vi "NI_Read XLSX File (revised, faster).vi"(4 "Remove empty rows":bool, 6 "Remove empty columns":bool, 8 "error in":errorcluster, 9 "Repeat multicell values":bool, 11 "XLSX File":path) -> (0 "error out":errorcluster, 2 "Sheet Names":string[](array[string]), 3 "Sheet Data":cluster{"Array":string[][]}[](array[cluster]))   [LabVIEW 2021, in "Files.lvlib"]
doc: "Reads all sheets from the specified <b>XLSX File</b>. This VI does <b>not</b> require Microsoft Excel to be installed.\n\nEach sheet is returned as a 2D Array of Strings. You will need to perform additional conversion if you require data in numeric format.\n\nTime data (date and/or time) is returned as a number of days elapsed since January 1, 1900. Hour/minute/second information will be returned as a fraction of a day (24 hours).\n\nAdded: option to fill table with repeated values to reflect multicell-spanning super-cells"
uses:
  Files.lvlib
  <vilib>/zip/NI_Unzip.lvlib
panel:
  out "UnDot?":bool
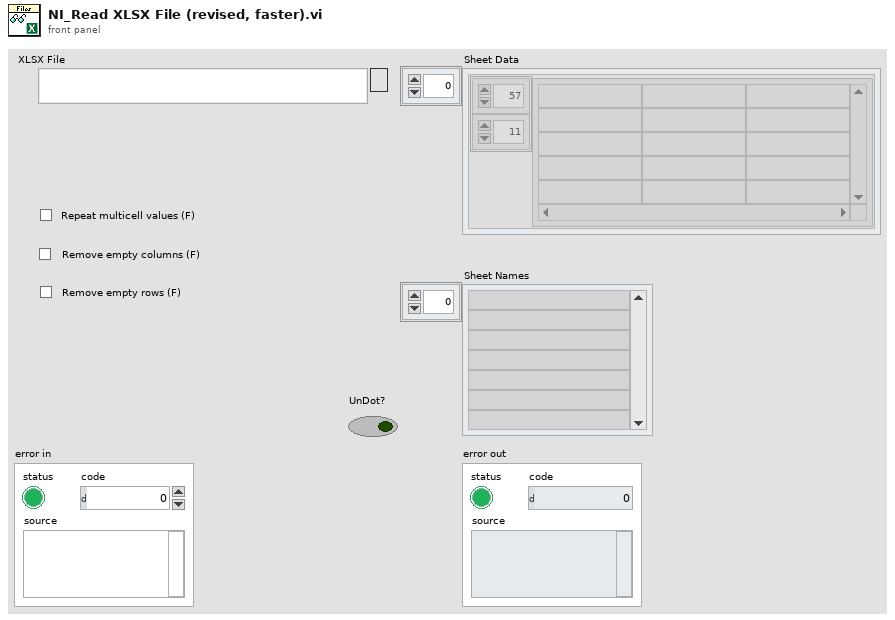
[diagram p1: front panel]
types:
  T1 = cluster{"Top Left Row":i32, "Top Left Col":i32, "Bottom Right Row":i32, "Bottom Right Col":i32}[]
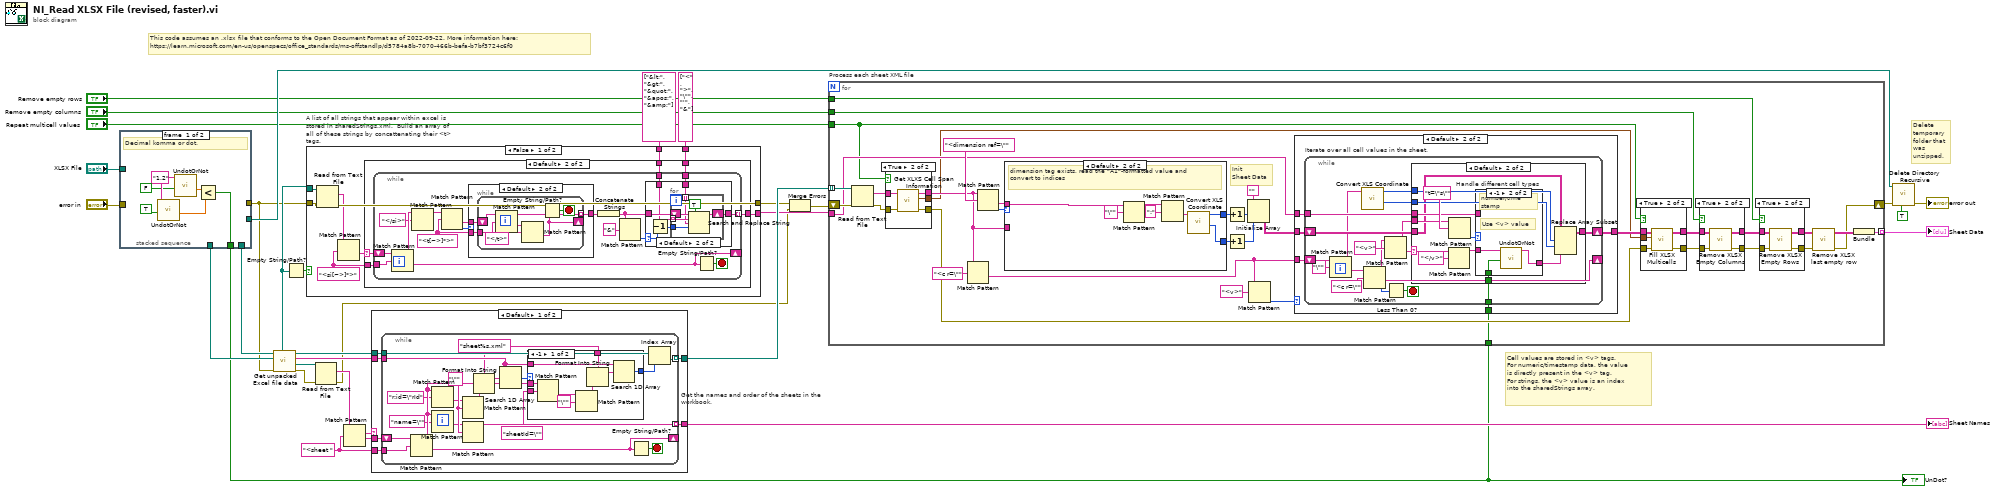
[diagram p0: block diagram]
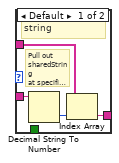
[diagram p8: hidden frame]
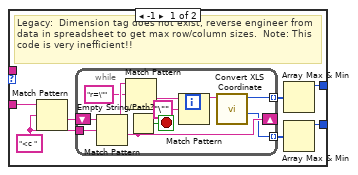
[diagram p9: hidden frame]
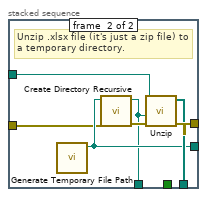
[diagram p16: hidden frame]
diagram:
  w27 = "<sheet "
  # "Cell values are stored in <v> tags.\nFor numeric/timestamp data, the value\nis directly present in the <v> tag.\nFor strings, the <v> value is an index\ninto the sharedStrings array."
  # "Delete temporary folder that was unzipped."
  # "This code assumes an .xlsx file that conforms to the Open Document Format as of 2022-09-22. More information here:\nhttps://learn.microsoft.com/en-us/openspecs/office_standards/ms-offstandlp/d5784a8b-7070-466b-befa-b7bf3724c6f0"
  n1 = stacked-sequence {
    tunnel: [_ w44] -> w4
    tunnel: [_ w43] -> w24
    tunnel: [_ w42] -> w31
    tunnel: [_ w41] -> w25
    tunnel: [w35 _] -> w10
    tunnel: "error in" -> [_ w40]
    tunnel: "XLSX File" -> [_ w39]
    frame #0 {
      w38 = "1.2" ("DottedNumber")
      # "Decimal komma or dot."
      n2 = call "UndotOrNot.vi"("UnDot?"=TRUE, "DottedNumber"=w38) -> ("Number"=w36:dbl)  [unwired: 8 in, 1 out]
      n3 = call "UndotOrNot.vi"("UnDot?"=FALSE, "DottedNumber"=w38) -> ("Number"=w37:dbl)  [unwired: 8 in, 1 out]
      n4 = Less?(x=w37, y=w36) -> (x < y?=w35:bool)
    }
    frame #1 {
      # "Unzip .xlsx file (it's just a zip file) to a temporary directory."
      n5 = call <vilib>:"Generate Temporary File Path.vi"() -> ("Unique Temporary File Path"=w42:path)  [unwired: 10 in, 1 out]
      n6 = call <vilib>:"Create Directory Recursive.vi"("error in (no error)"=w40, "directory"=w42) -> ("error out"=w45:errorcluster, "directory copy"=w41:path)  [unwired: 3 in, 1 out]
      n7 = call <vilib>:"Unzip.vi"("error in (no error)"=w45, "Target directory (same as Zip file if empty)"=w41, "Zip file"=w39) -> ("error out"=w44:errorcluster, "Unzipped files"=w43:path[])  [unwired: 6 in, 1 out]
    }
  }
  "UnDot?" <- w10
  n8 = call "Get unpacked Excel file data.vi"("Error In"=w4, "temp zip path"=w25, "Unzipped files"=w24) -> ("Error Out"=w3:errorcluster, "workbook.xml path"=w5:path, "sheet file names"=w6:string[], "sheet paths"=w26:path[], "sharedStrings path"=w15:path)  [unwired: 4 in]
  n9 = Empty String/Path?(string/path=w15) -> (empty?=w16:bool)
  n10 = case "A list of all strings that appear within excel is stored in sharedStrings.xml.  Build an array of all of these strings by concattenating their <t> tags." shown="False" w16 {
    tunnel: w4 -> [w54 w100]
    tunnel: [w52 w100] -> w18
    tunnel: w15 -> [w53 _]
    tunnel: [w51 _] -> w17
    tunnel: string[] ["&lt;", "&gt;", "&quot;", "&apos;", "&amp;"] -> [w47 _]
    tunnel: string[] ["<", ">", "\"", "'", "&"] -> [w46 _]
    frame False {
      w49 = "<si[~>]*>" ("regular expression")
      n11 = Read from Text File(file (use dialog)=w53, error in=w54) -> (text=w48:string, error out=w52:errorcluster)  [unwired: 2 in, 2 out]
      n12 = Match Pattern(string=w48, regular expression=w49) -> (after substring=w50:string)  [unwired: 1 in, 3 out]
      n13 = case shown="Default" w50 {
        selector: w50 -> [_ w57]
        tunnel: [_ w59] -> w51
        tunnel: w49 -> [_ w58]
        tunnel: w47 -> [_ w56]
        tunnel: w46 -> [_ w55]
        frame "" {
        }
        frame Default {
          n14 = while {
            tunnel: [w63] -> w59 mode=indexing
            tunnel: w58 -> [w75]
            shift-right: [w67] -> _
            shift-left: w57 -> [w69]
            tunnel: w56 -> [w61]
            tunnel: w55 -> [w60]
            stop <- w66 stop-if-true
            w68 = "<t[~>]*>" ("regular expression")
            n15 = Match Pattern(string=w69, regular expression=w75) -> (before substring=w74:string, after substring=w67:string)  [unwired: 1 in, 2 out]
            n16 = Match Pattern(string=w74, regular expression="</si>") -> (before substring=w71:string)  [unwired: 1 in, 3 out]
            n17 = Match Pattern(string=w71, regular expression=w68) -> (after substring=w70:string, offset past match=w72:i32)  [unwired: 1 in, 2 out]
            n18 = case shown="Default" w72 {
              tunnel: [_ w92] -> w76
              tunnel: w68 -> [_ w91]
              tunnel: w70 -> [_ w90]
              frame -1 {
              }
              frame Default {
                n19 = while {
                  tunnel: [w93] -> w92 mode=indexing
                  tunnel: w91 -> [w99]
                  shift-right: [w96] -> _
                  shift-left: w90 -> [w98]
                  stop <- w95 stop-if-true
                  n20 = Match Pattern(string=w98, regular expression="</t>") -> (before substring=w93:string, after substring=w97:string)  [unwired: 1 in, 2 out]
                  n21 = Match Pattern(string=w97, regular expression=w99) -> (after substring=w96:string)  [unwired: 1 in, 3 out]
                  n22 = Empty String/Path?(string/path=w96) -> (empty?=w95:bool)
                }
              }
            }
            n23 = Concatenate Strings(w76) -> (w62:string)
            n24 = Match Pattern(string=w62, regular expression="&") -> (offset past match=w64:i32)  [unwired: 1 in, 3 out]
            n25 = case shown="Default" w64 {
              selector: w64 -> [_ w79]
              tunnel: w62 -> [w77 w82]
              tunnel: [w77 w83] -> w63
              tunnel: w61 -> [_ w81]
              tunnel: w60 -> [_ w80]
              frame -1 {
              }
              frame Default {
                n26 = Decrement(x=w79) -> (x-1=w78:i32)
                n27 = for {
                  shift-right: [w88] -> w83
                  shift-left: w82 -> [w89]
                  tunnel: w81 -> [w86] mode=indexing
                  tunnel: w80 -> [w85] mode=indexing
                  tunnel: w78 -> [w84]
                  n28 = Search and Replace String(replace all?=TRUE ("replace all? (F)"), input string=w89, search string=w86, replace string=w85, offset=w84) -> (result string=w88:string)  [unwired: 3 in, 3 out]
                }
              }
            }
            n29 = Empty String/Path?(string/path=w67) -> (empty?=w66:bool)
          }
        }
      }
    }
    frame True {
      # "No sharedStrings.xml file within .xlsx."
    }
  }
  n30 = Read from Text File(file (use dialog)=w5, error in=w3) -> (text=w28:string, error out=w1:errorcluster)  [unwired: 2 in, 2 out]
  n31 = Match Pattern(string=w28, regular expression=w27) -> (match substring=w23:string, after substring=w22:string)  [unwired: 1 in, 2 out]
  n32 = case shown="Default" w23 {
    tunnel: [w106 _] -> w29
    tunnel: w27 -> [w105 _]
    tunnel: [w104 _] -> w21
    tunnel: w26 -> [w103 _]
    tunnel: w6 -> [w102 _]
    tunnel: w22 -> [w101 _]
    frame Default {
      n33 = while "Get the names and order of the sheets in the workbook." {
        tunnel: [w126] -> w106 mode=indexing
        tunnel: w102 -> [w122]
        tunnel: w103 -> [w120]
        tunnel: [w118] -> w104 mode=indexing
        tunnel: w105 -> [w115]
        shift-right: [w108] -> _
        shift-left: w101 -> [w109]
        stop <- w107 stop-if-true
        w117 = "sheet%s.xml" ("format string")
        w125 = "\"" ("regular expression")
        n34 = Match Pattern(string=w109, regular expression=w115) -> (before substring=w112:string, after substring=w108:string)  [unwired: 1 in, 2 out]
        n35 = Match Pattern(string=w112, regular expression="r:id=\"rId") -> (after substring=w114:string)  [unwired: 1 in, 3 out]
        n36 = Match Pattern(string=w112, regular expression="name=\"") -> (after substring=w113:string)  [unwired: 1 in, 3 out]
        n37 = Match Pattern(string=w114, regular expression=w125) -> (before substring=w124:string)  [unwired: 1 in, 3 out]
        n38 = Match Pattern(string=w113, regular expression=w125) -> (before substring=w126:string)  [unwired: 1 in, 3 out]
        n39 = Format Into String(format string=w117, w124) -> (resulting string=w123:string)  [unwired: 2 in, 1 out]
        n40 = Search 1D Array(1D array=w122, element=w123) -> (index of element=w121:i32)  [unwired: 1 in]
        n41 = case shown="-1" w121 {
          selector: w121 -> [_ w136]
          tunnel: w122 -> [w133 _]
          tunnel: [w131 w136] -> w119
          tunnel: w117 -> [w130 _]
          tunnel: "sheetId=\"" ("regular expression") -> [w129 _]
          tunnel: w112 -> [w128 _]
          frame -1 {
            n42 = Match Pattern(string=w128, regular expression=w129) -> (after substring=w127:string)  [unwired: 1 in, 3 out]
            n43 = Match Pattern(string=w127, regular expression="\"") -> (before substring=w135:string)  [unwired: 1 in, 3 out]
            n44 = Format Into String(format string=w130, w135) -> (resulting string=w134:string)  [unwired: 2 in, 1 out]
            n45 = Search 1D Array(1D array=w133, element=w134) -> (index of element=w131:i32)  [unwired: 1 in]
          }
          frame Default {
          }
        }
        n46 = Empty String/Path?(string/path=w108) -> (empty?=w107:bool)
        n47 = Index Array(array=w120, index=w119) -> (element=w118:path)
      }
    }
    frame "" {
    }
  }
  "Sheet Names" <- w29
  n48 = Merge Errors(w18, w1) -> (w2:errorcluster)
  n49 = for "Process each sheet XML file" {
    shift-right: [w137] -> w19
    shift-left: w2 -> [w171]
    tunnel: w21 -> [w170] mode=indexing
    tunnel: [w165] -> w20 mode=indexing
    tunnel: w17 -> [w164]
    tunnel: w10 -> [w148]
    tunnel: "Repeat multicell values" -> [w147]
    tunnel: "Remove empty columns" -> [w144]
    tunnel: "Remove empty rows" -> [w143]
    # "Init\nSheet Data"
    n50 = Read from Text File(file (use dialog)=w170, error in=w171) -> (text=w155:string, error out=w153:errorcluster)  [unwired: 2 in, 2 out]
    n51 = case shown="True" w147 {
      tunnel: w155 -> [w192 w197]
      tunnel: [w192 w196] -> w154
      tunnel: w153 -> [w191 w195]
      tunnel: [_ w194] -> w151
      tunnel: [w191 w193] -> w150
      frame False {
      }
      frame True {
        n52 = call "Get XLXS Cell Span Information.vi"("Error In"=w195, "String"=w197) -> ("Error Out"=w193:errorcluster, "Cell Span"=w194:T1, "String dup"=w196:string)  [unwired: 7 in]
      }
    }
    n53 = Match Pattern(string=w154, regular expression="<c r=\"") -> (after substring=w149:string)  [unwired: 1 in, 3 out]
    n54 = Match Pattern(string=w154, regular expression="<dimension ref=\"") -> (after substring=w168:string, offset past match=w161:i32)  [unwired: 1 in, 2 out]
    n55 = case shown="Default" w161 {
      tunnel: w168 -> [_ w267]
      tunnel: [w247 w262] -> w163
      tunnel: [w246 w261] -> w162
      tunnel: w154 -> [w245 _]
      frame -1 {
        w243 = "<c " ("regular expression")
        # "Legacy:  Dimension tag does not exist, reverse engineer from data in spreadsheet to get max row/column sizes.  Note: This code is very inefficient!!"
        n56 = Match Pattern(string=w245, regular expression=w243) -> (after substring=w244:string)  [unwired: 1 in, 3 out]
        n57 = while {
          tunnel: [w250] -> w249 mode=indexing
          tunnel: [w259] -> w248 mode=indexing
          tunnel: w243 -> [w255]
          shift-right: [w252] -> _
          shift-left: w244 -> [w254]
          stop <- w251 stop-if-true
          n58 = Match Pattern(string=w254, regular expression=w255) -> (before substring=w257:string, after substring=w252:string)  [unwired: 1 in, 2 out]
          n59 = Match Pattern(string=w257, regular expression="r=\"") -> (after substring=w256:string)  [unwired: 1 in, 3 out]
          n60 = Empty String/Path?(string/path=w252) -> (empty?=w251:bool)
          n61 = Match Pattern(string=w256, regular expression="\"") -> (before substring=w258:string)  [unwired: 1 in, 3 out]
          n62 = call "Convert XLS Coordinate.vi"("Excel coordinate"=w258) -> ("Column"=w250:i32, "Row"=w259:i32)  [unwired: 9 in]
        }
        n63 = Array Max & Min(array=w248) -> (max value=w247:i32)  [unwired: 3 out]
        n64 = Array Max & Min(array=w249) -> (max value=w246:i32)  [unwired: 3 out]
      }
      frame Default {
        # "Code copied from:\n[LabVIEW 20xx]\\vi.lib\\addons\\_office\\excel.llb\\Excel Get Excel Location.vi"
        # "dimension tag exists, read the \"A1\"-formatted value and convert to indices"
        n65 = Match Pattern(string=w267, regular expression="\"") -> (before substring=w265:string)  [unwired: 1 in, 3 out]
        n66 = Match Pattern(string=w265, regular expression=":") -> (after substring=w263:string)  [unwired: 1 in, 3 out]
        n67 = call "Convert XLS Coordinate.vi"("Excel coordinate"=w263) -> ("Column"=w261:i32, "Row"=w262:i32)  [unwired: 9 in]
      }
    }
    n68 = Increment(x=w163) -> (x+1=w160:i32)
    n69 = Increment(x=w162) -> (x+1=w159:i32)
    n70 = Initialize Array("", w160, w159) -> (w166:string[][])
    n71 = Match Pattern(string=w149, regular expression="<v>") -> (offset past match=w156:i32)  [unwired: 1 in, 3 out]
    n72 = case shown="Default" w156 {
      tunnel: w166 -> [w198 w203]
      tunnel: [w198 w202] -> w152
      tunnel: w164 -> [_ w201]
      tunnel: w149 -> [_ w200]
      tunnel: w148 -> [_ w199]
      frame -1 {
        # "No content, so skip"
      }
      frame Default {
        n73 = while "Iterate over all cell values in the sheet." {
          shift-right: [w221] -> w202
          shift-left: w203 -> [w220]
          tunnel: w201 -> [w219]
          shift-right: [w211] -> _
          shift-left: w200 -> [w217]
          tunnel: w199 -> [w204]
          stop <- w209 stop-if-true
          n74 = Match Pattern(string=w217, regular expression="\"") -> (before substring=w216:string, after substring=w212:string)  [unwired: 1 in, 2 out]
          n75 = call "Convert XLS Coordinate.vi"("Excel coordinate"=w216) -> ("Column"=w214:i32, "Row"=w215:i32)  [unwired: 9 in]
          n76 = Match Pattern(string=w212, regular expression="<c r=\"") -> (before substring=w206:string, after substring=w211:string, offset past match=w210:i32)  [unwired: 1 in, 1 out]
          n77 = Match Pattern(string=w206, regular expression="<v>") -> (before substring=w207:string, after substring=w205:string)  [unwired: 1 in, 2 out]
          n78 = Less Than 0?(x=w210) -> (x < 0?=w209:bool)
          n79 = case shown="Default" w205 {
            selector: w205 -> [_ w225]
            tunnel: [w222 w235] -> w221
            tunnel: w220 -> [w222 w224]
            tunnel: w219 -> [_ w229]
            tunnel: w207 -> [_ w228]
            tunnel: w215 -> [_ w227]
            tunnel: w214 -> [_ w226]
            tunnel: w204 -> [_ w223]
            frame "" {
              # "Empty field or STOP=T, so skip"
            }
            frame Default {
              n80 = Match Pattern(string=w225, regular expression="</v>") -> (before substring=w230:string)  [unwired: 1 in, 3 out]
              n81 = Match Pattern(string=w228, regular expression="t=\"s\"") -> (offset past match=w232:i32)  [unwired: 1 in, 3 out]
              n82 = case "Handle different cell types" shown="-1" w232 {
                tunnel: [w237 w241] -> w231
                tunnel: w230 -> [w239 w242]
                tunnel: w229 -> [w236 _]
                tunnel: w223 -> [_ w240]
                frame Default {
                  # "Pull out sharedString\nat specified index"
                  # "string"
                  n83 = Decimal String To Number(string=w239) -> (number=w238:i32)  [unwired: 2 in, 1 out]
                  n84 = Index Array(array=w236, index=w238) -> (element=w237:string)
                }
                frame -1 {
                  # "Use <v> value"
                  # "number/time stamp"
                  n85 = call "UndotOrNot.vi"("UnDot?"=w240, "DottedNumber"=w242) -> ("result string"=w241:string)  [unwired: 8 in, 1 out]
                }
              }
              n86 = Replace Array Subset(array=w224, new element=w231, index (row)=w227, index (col)=w226) -> (w235:string[][])
            }
          }
        }
      }
    }
    n87 = case shown="True" w147 {
      tunnel: w152 -> [w185 w190]
      tunnel: [w185 w189] -> w145
      tunnel: w151 -> [_ w188]
      tunnel: w150 -> [w184 w187]
      tunnel: [w184 w186] -> w146
      frame False {
      }
      frame True {
        n88 = call "Fill XLSX Multicells.vi"("error in (no error)"=w187, "Cell Span"=w188, "Array in"=w190) -> ("error out"=w186:errorcluster, "Array out"=w189:string[][])  [unwired: 7 in]
      }
    }
    n89 = case shown="True" w144 {
      tunnel: [w179 w183] -> w142
      tunnel: [w178 w182] -> w141
      tunnel: w146 -> [w178 w181]
      tunnel: w145 -> [w179 w180]
      frame False {
      }
      frame True {
        n90 = call "Remove XLSX Empty Columns.vi"("error in (no error)"=w181, "Array in"=w180) -> ("error out"=w182:errorcluster, "Array out"=w183:string[][])  [unwired: 7 in, 1 out]
      }
    }
    n91 = case shown="True" w143 {
      tunnel: [w173 w177] -> w139
      tunnel: [w172 w176] -> w138
      tunnel: w141 -> [w172 w175]
      tunnel: w142 -> [w173 w174]
      frame False {
      }
      frame True {
        n92 = call "Remove XLSX Empty Rows.vi"("error in (no error)"=w175, "Array in"=w174) -> ("error out"=w176:errorcluster, "Array out"=w177:string[][])  [unwired: 7 in, 1 out]
      }
    }
    n93 = call "Remove XLSX last empty row.vi"("Error In"=w138, "Array in"=w139) -> ("Error Out"=w137:errorcluster, "Array out"=w140:string[][])  [unwired: 7 in, 1 out]
    n94 = Bundle("Array out"=w140) -> (w165:cluster{"Array out":string[][]})  [unwired: 1 in]
  }
  "Sheet Data" <- w20
  n95 = call <vilib>:"Delete Directory Recursive.vi"("keep deleting on error? (F)"=TRUE, "error in (no error)"=w19, "Folder to Delete"=w31) -> ("error out"=→"error out":errorcluster)  [unwired: 7 in, 1 out]
